vi "simpleInterpreter2.vi"() -> ()   [LabVIEW 2011]
uses:
  <vilib>/Utility/inputDevices.llb/keyboardAcquire.vi
  lib/labviewwait.dll
panel:
  out "lua_type":i32(ring) items=["LUA_TNONE"=-1, "LUA_TNIL"=0, "LUA_TBOOLEAN"=1, "LUA_TLIGHTUSERDATA"=2, "LUA_TNUMBER "=3, "LUA_TSTRING"=4, "LUA_TTABLE"=5, "LUA_TFUNCTION"=6, "LUA_TUSERDATA"=7, "LUA_TTHREAD"=8, "LUA_NUMTAGS "=9]
  out "lua_State *commandthread":u64
  out "lua_State *L":u64
  out "lua_State *print thread":u64
  in  "status refrash":bool
  in  "command refrash":bool
  out "stack":i32
  out "LoadBufferStatus":i32(ring) items=["LUA_OK", "LUA_YIELD", "LUA_ERRRUN", "LUA_ERRSYNTAX", "LUA_ERRMEM", "LUA_ERRGCMM", "LUA_ERRERR"]
  out "PcallStatus":i32(ring) items=["LUA_OK", "LUA_YIELD", "LUA_ERRRUN", "LUA_ERRSYNTAX", "LUA_ERRMEM", "LUA_ERRGCMM", "LUA_ERRERR"]
  in  "停止":bool
  in  "command(ctrl+enter)":string
  out "status":string
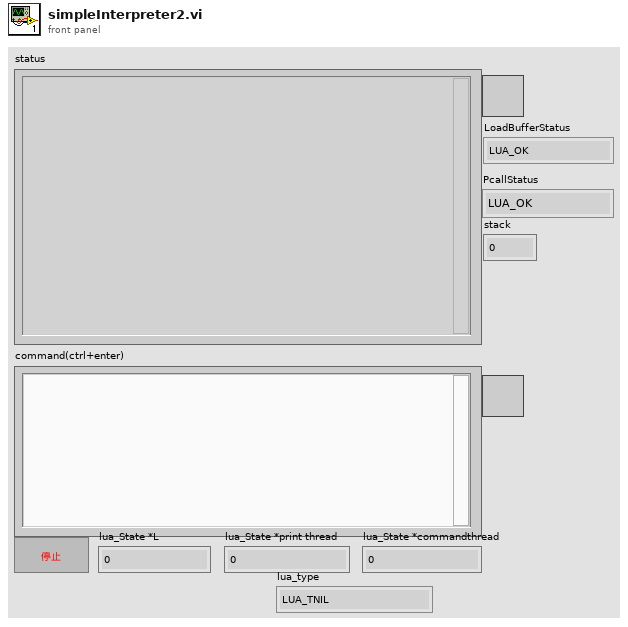
[diagram p1: front panel]
types:
  T1 = enum16{"0", "1", "2", "3", "4", "5", "6", "7", "8", "9", "A", "B", "C", "D", "E", "F", "G", "H", "I", "J", "K", "L", "M", "N", "O", "P", "Q", "R", "S", "T", "U", "V", "W", "X", "Y", "Z", "F1", "F2", "F3", "F4", "F5", "F6", "F7", "F8", "F9", "F10", "F11", "F12", "F13", "F14", "F15", "ADD", "BACK", "BACKSLASH", "CAPITAL", "COMMA", "DECIMAL", "DELETE", "DIVIDE", "DOWN", "END", "EQUALS", "ESCAPE", "GRAVE (`)", "HOME", "INSERT", "LBRACKET", "LCONTROL", "LEFT", "L ALT", "LSHIFT", "LWIN", "MINUS", "MULTIPLY", "NEXT", "NUMLOCK", "NUMPAD_0", "NUMPAD_1", "NUMPAD_2", "NUMPAD_3", "NUMPAD_4", "NUMPAD_5", "NUMPAD_6", "NUMPAD_7", "NUMPAD_8", "NUMPAD_9", "PAUSE", "PERIOD", "PRIOR (PG UP)", "RBRACKET", "RCONTROL", "RETURN", "RIGHT", "R ALT", "RSHIFT", "RWIN", "SCROLL", "SEMICOLON", "SLASH", "SPACE", "SUBTRACT", "TAB", "UP", "ENTER (num pad)", "' (quote)"}[]
  T2 = enum16{"0", "1", "2", "3", "4", "5", "6", "7", "8", "9", "A", "B", "C", "D", "E", "F", "G", "H", "I", "J", "K", "L", "M", "N", "O", "P", "Q", "R", "S", "T", "U", "V", "W", "X", "Y", "Z", "F1", "F2", "F3", "F4", "F5", "F6", "F7", "F8", "F9", "F10", "F11", "F12", "F13", "F14", "F15", "ADD", "BACK", "BACKSLASH", "CAPITAL", "COMMA", "DECIMAL", "DELETE", "DIVIDE", "DOWN", "END", "EQUALS", "ESCAPE", "GRAVE (`)", "HOME", "INSERT", "LBRACKET", "LCONTROL", "LEFT", "L ALT", "LSHIFT", "LWIN", "MINUS", "MULTIPLY", "NEXT", "NUMLOCK", "NUMPAD_0", "NUMPAD_1", "NUMPAD_2", "NUMPAD_3", "NUMPAD_4", "NUMPAD_5", "NUMPAD_6", "NUMPAD_7", "NUMPAD_8", "NUMPAD_9", "PAUSE", "PERIOD", "PRIOR (PG UP)", "RBRACKET", "RCONTROL", "RETURN", "RIGHT", "R ALT", "RSHIFT", "RWIN", "SCROLL", "SEMICOLON", "SLASH", "SPACE", "SUBTRACT", "TAB", "UP", "ENTER (num pad)", "' (quote)"}
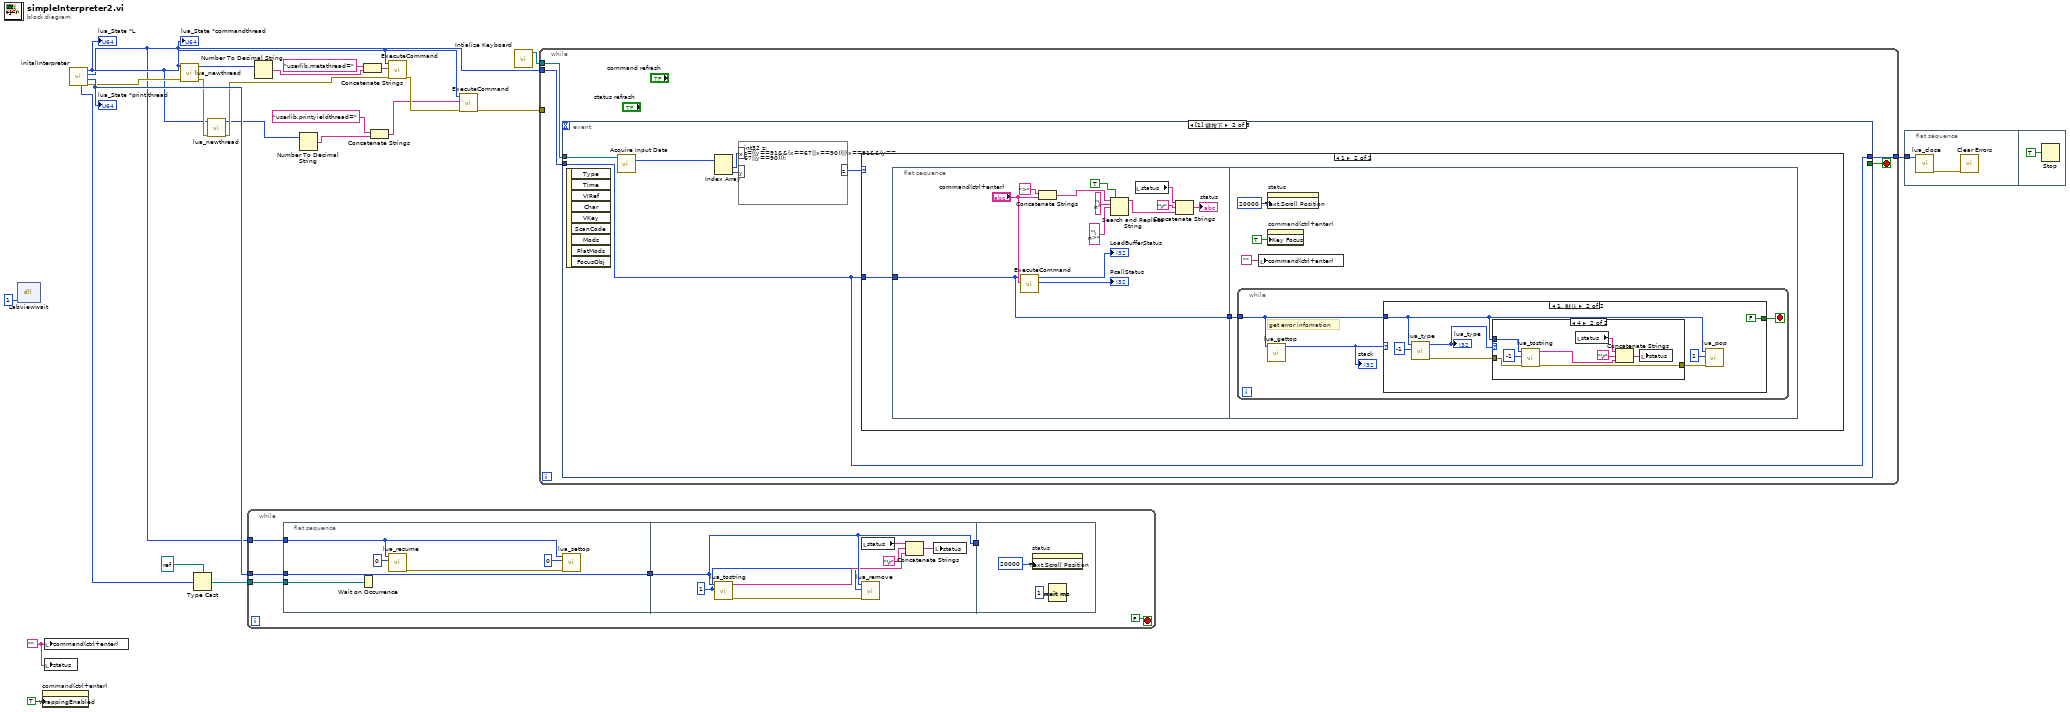
[diagram p0: block diagram]
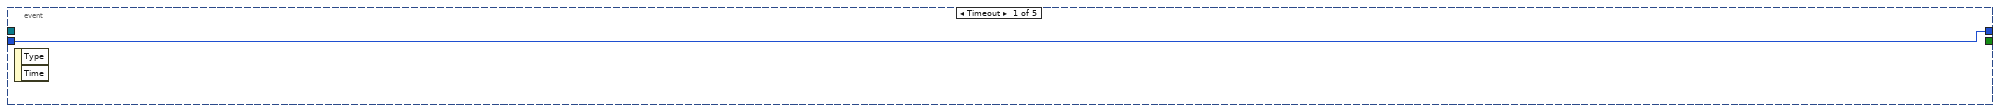
[diagram p2: hidden frame]
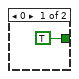
[diagram p4: hidden frame]
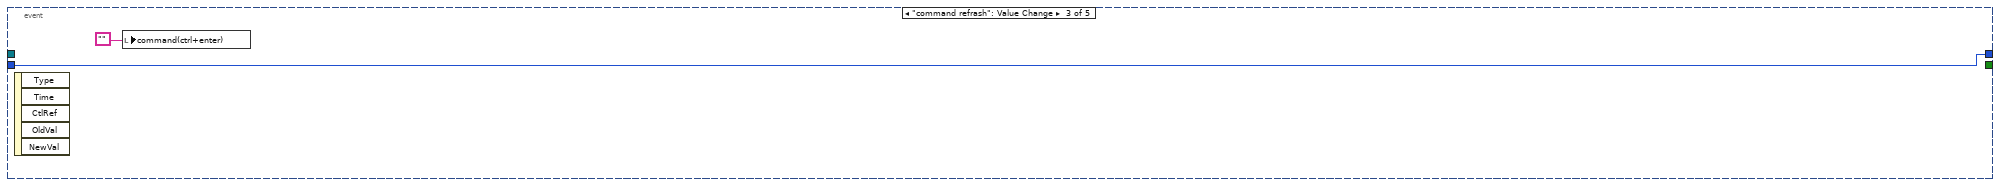
[diagram p6: hidden frame]
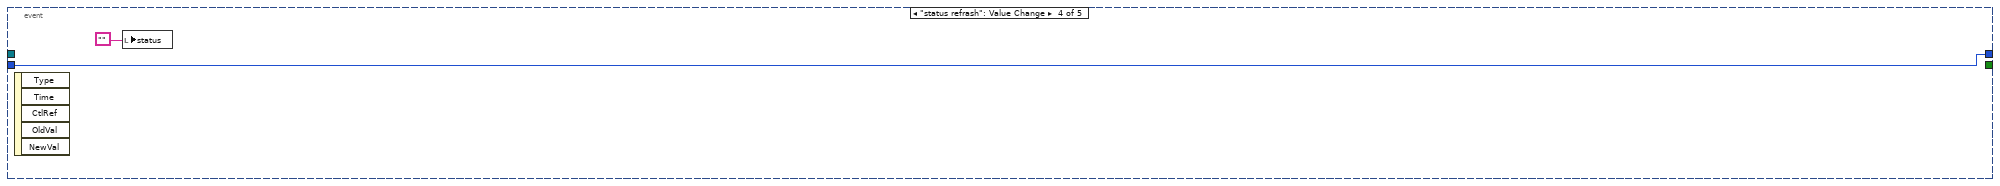
[diagram p7: hidden frame]
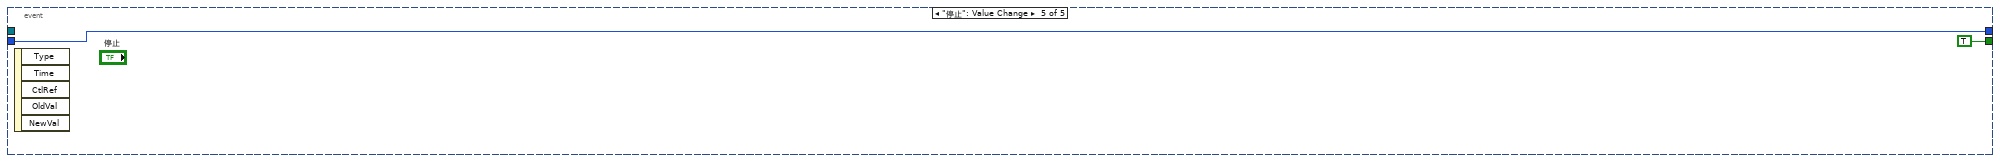
[diagram p8: hidden frame]
diagram:
  w24 = ""
  n1 = dll-call lib="G:/My DBank/_work_pan/LuaDllToLabview/lib/labviewwait.dll" fn="Labviewwait"("wait"=1) -> ()  [unwired: 5 in, 2 out]
  n2 = property on="command(ctrl+enter)" class="Str"("WrappingEnabled"=TRUE ("启用自动换行")) -> ()  [unwired: 2 in, 2 out]
  n3 = local write "command(ctrl+enter)"(w24) -> ()
  n4 = local write "status"(w24) -> ()
  n5 = call "initalInterpreter.vi"() -> ("错误输出"=w9:errorcluster, "lua_State *print thread"=w17:u64, "lua_State *commandthread"=w2:u64, "lua_State *mainthread"=w4:u64, "printoccur"=w18:i32)  [unwired: 5 in, 2 out]
  "lua_State *print thread" <- w17
  "lua_State *L" <- w4
  "lua_State *commandthread" <- w2
  n6 = call "lua_newthread.vi"("error in"=w9, "lua_State *L"=w4) -> ("error out"=w8:errorcluster, "lua_State *lua_newthread"=w14:u64)  [unwired: 8 in]
  n7 = Type Cast(type=refnum<k4> refnum ("事件发生"), x=w18) -> (*(type *) &x=w19:refnum<k4>)
  n8 = call "lua_newthread.vi"("error in"=w8, "lua_State *L"=w4) -> ("error out"=w7:errorcluster, "lua_State *lua_newthread"=w3:u64)  [unwired: 8 in]
  n9 = while {
    tunnel: w17 -> [w29]
    tunnel: w19 -> [w26]
    tunnel: w2 -> [w25]
    stop <- FALSE stop-if-true
    n10 = flat-sequence {
      tunnel: w29 -> [w36]
      tunnel: [w36] -> w27
      tunnel: w26 -> [w35]
      tunnel: w25 -> [w33]
      tunnel: [w43] -> w28
      tunnel: w27 -> [w43]
      tunnel: w28 -> [_]
      frame #0 {
        n11 = Wait on Occurrence(2:w35) -> ()  [unwired: 2 in, 1 out]
        n12 = call "lua_resume.vi"("int nargs"=0, "lua_State *L"=w33) -> ("error out"=w31:errorcluster)  [unwired: 9 in]
        n13 = call "lua_settop.vi"("error in"=w31, "index"=0, "lua_State *L"=w33) -> ()  [unwired: 8 in, 1 out]
      }
      frame #1 {
        w37 = 1 ("index")
        n14 = call "lua_tostring.vi"("index"=w37, "lua_State *L"=w43) -> ("error out"=w38:errorcluster, "constant string"=w39:string)  [unwired: 8 in]
        n15 = local read "status"() -> (w41:string)
        n16 = call "lua_remove.vi"("error in"=w38, "int index"=w37, "lua_State *L"=w43) -> ()  [unwired: 8 in, 1 out]
        n17 = Concatenate Strings(w41, "\r", w39) -> (w42:string)
        n18 = local write "status"(w42) -> ()
      }
      frame #2 {
        n19 = property on="status" class="Str"("Text.Scroll Position"=u32 20000 ("文本.滚动条位置")) -> ()  [unwired: 2 in, 2 out]
        n20 = Wait (ms)(milliseconds to wait=u32 1 ("等待时间（毫秒）")) -> ()  [unwired: 1 out]
      }
    }
  }
  n21 = Number To Decimal String(number=w14) -> (decimal integer string=w16:string)  [unwired: 1 in]
  n22 = Number To Decimal String(number=w3) -> (decimal integer string=w6:string)  [unwired: 1 in]
  n23 = Concatenate Strings("userlib.metathread=" ("字符串"), w16) -> (w13:string)
  n24 = Concatenate Strings("userlib.printyieldthread=" ("字符串"), w6) -> (w5:string)
  n25 = call "ExecuteCommand.vi"("error in"=w7, "command(ctrl+enter)"=w13, "lua_State *luaL_newstate"=w4) -> ("error out"=w12:errorcluster)  [unwired: 6 in, 2 out]
  n26 = call "ExecuteCommand.vi"("error in"=w12, "command(ctrl+enter)"=w5, "lua_State *luaL_newstate"=w4) -> ("error out"=w11:errorcluster)  [unwired: 6 in, 2 out]
  n27 = call <vilib>:"Intialize Keyboard.vi"() -> ("device ID"=w22:refnum<k1>)  [unwired: 10 in, 1 out]
  n28 = while {
    tunnel: w2 -> [w49]
    tunnel: [w47] -> w21
    tunnel: w22 -> [w46]
    tunnel: w11 -> [_]
    stop <- w48 stop-if-true
    n29 = event shown="[1] 键按下" {
      selector: _ -> [_ _ _ _ _]
      dyn-events: _ -> [_ _ _ _ _]
      timeout: _ -> [_ _ _ _ _]
      tunnel: w49 -> [w50 w51 w96 w98 w100]
      tunnel: [_ _ _ _ TRUE ("停止 2")] -> w48
      tunnel: [w50 w51 w96 w98 w100] -> w47
      tunnel: w46 -> [_ w56 _ _ _]
      event Timeout {
        n30 = event-data() -> ()  [unwired: 1 in, 2 out]
      }
      event Key Down {
        n31 = event-data() -> ()  [unwired: 1 in, 9 out]
        n32 = call-poly <vilib>:"Acquire Input Data.vi"("device ID"=w56) -> ("keys pressed"=w55:T1)  [unwired: 16 in, 2 out]
        n33 = Index Array(array=w55) -> (element #1=w54:T2, element #2=w53:T2)  [unwired: 2 in]
        n34 = formula code="int32 z;\nz=((y==91&&(x==67||x==90))||(x==91&&(y==67||y==90)));"("x"=w54, "y"=w53) -> ("z"=w52:i32)
        n35 = case shown="1" w52 {
          tunnel: w51 -> [_ w58]
          frame 0, Default {
          }
          frame 1 {
            n36 = flat-sequence {
              tunnel: w58 -> [w59]
              tunnel: [w59] -> w57
              tunnel: w57 -> [w72]
              frame #0 {
                n37 = call "ExecuteCommand.vi"("command(ctrl+enter)"="command(ctrl+enter)", "lua_State *luaL_newstate"=w59) -> ("thread status 2"=→"PcallStatus":i32, "thread status"=→"LoadBufferStatus":i32)  [unwired: 7 in, 1 out]
                n38 = Concatenate Strings(">", "command(ctrl+enter)") -> (w64:string)
                n39 = Search and Replace String(replace all?=TRUE ("替换全部？(F)"), input string=w64, search string="\n" ("搜索字符串"), replace string="\n>" ("替换字符串(\"\")")) -> (result string=w60:string)  [unwired: 4 in, 3 out]
                n40 = local read "status"() -> (w70:string)
                n41 = Concatenate Strings(w70, "\r", w60) -> (→"status":string)
              }
              frame #1 {
                n42 = while {
                  tunnel: w72 -> [w77]
                  stop <- w76 stop-if-true
                  # "get error infomation"
                  n43 = call "lua_gettop.vi"("lua_State *L"=w77) -> ("lua_gettop"=w78:i32)  [unwired: 9 in, 1 out]
                  "stack" <- w78
                  n44 = case shown="1, 默认" w78 {
                    tunnel: w77 -> [_ w83]
                    tunnel: [TRUE FALSE] -> w76
                    frame 0 {
                    }
                    frame 1, Default {
                      n45 = call "lua_type.vi"("int index"=-1, "lua_State *L"=w83) -> ("error out"=w85:errorcluster, "lua_type"=w80:i32)  [unwired: 8 in]
                      "lua_type" <- w80
                      n46 = case shown="4" w80 {
                        tunnel: w85 -> [w87 w95]
                        tunnel: [w87 w94] -> w84
                        tunnel: w83 -> [_ w93]
                        frame 0, Default {
                        }
                        frame 4 {
                          n47 = call "lua_tostring.vi"("error in"=w95, "index"=-1, "lua_State *L"=w93) -> ("error out"=w94:errorcluster, "constant string"=w88:string)  [unwired: 7 in]
                          n48 = local read "status"() -> (w90:string)
                          n49 = Concatenate Strings(w90, "\r", w88) -> (w89:string)
                          n50 = local write "status"(w89) -> ()
                        }
                      }
                      n51 = call "lua_pop.vi"("error in"=w84, "n"=1, "lua_State *L"=w83) -> ()  [unwired: 8 in, 1 out]
                    }
                  }
                }
                n52 = local write "command(ctrl+enter)"("") -> ()
                n53 = property on="status" class="Str"("Text.Scroll Position"=u32 20000 ("文本.滚动条位置")) -> ()  [unwired: 2 in, 2 out]
                n54 = property on="command(ctrl+enter)" class="Str"("Key Focus"=TRUE ("键选中")) -> ()  [unwired: 2 in, 2 out]
              }
            }
          }
        }
      }
      event "command refrash": Value Change {
        n55 = event-data() -> ()  [unwired: 1 in, 5 out]
        n56 = local write "command(ctrl+enter)"("") -> ()
      }
      event "status refrash": Value Change {
        n57 = event-data() -> ()  [unwired: 1 in, 5 out]
        n58 = local write "status"("") -> ()
      }
      event "停止": Value Change {
        n59 = event-data() -> ()  [unwired: 1 in, 5 out]
      }
    }
  }
  n60 = flat-sequence {
    tunnel: w21 -> [w103]
    frame #0 {
      n61 = call "lua_close.vi"("lua_State *L"=w103) -> ("error out"=w102:errorcluster)  [unwired: 10 in]
      n62 = call <vilib>:"Clear Errors.vi"("error in (no error)"=w102) -> ()  [unwired: 6 in, 1 out]
    }
    frame #1 {
      n63 = Stop(stop? (T)=TRUE ("停止？(T)")) -> ()
    }
  }
